vi "Init.vi"(8 "error in (no error)":errorcluster, 9 "Logging Root":path, 10 "VolatusAPI":refnum<class "VolatusAPI.lvclass">, 11 "EventHandlerTask in":refnum<class "EventHandlerTask.lvclass">) -> (0 "error out":errorcluster, 3 "EventHandlerTask out":refnum<class "EventHandlerTask.lvclass">)   [LabVIEW 2020, in "Volatus.lvlib" / "EventHandlerTask.lvclass"]
uses:
  EventHandlerTask.lvclass
  EventHandlerTask.lvclass/EventHandlerTask.ctl
  VolatusAPI/VolatusAPI.lvclass
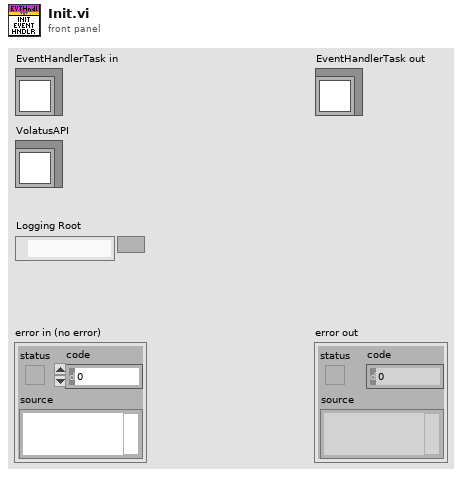
[diagram p1: front panel]
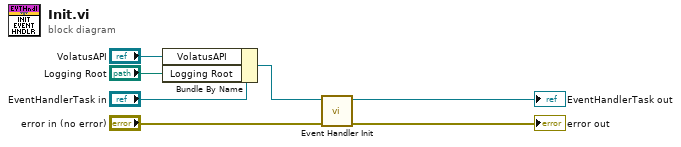
[diagram p0: block diagram]
diagram:
  n1 = Bundle By Name(cluster="EventHandlerTask in", "VolatusAPI"="VolatusAPI", "Logging Root"="Logging Root") -> (w2:refnum<class "EventHandlerTask.lvclass">)
  n2 = call-dynamic "Event Handler Init.vi"("error in (no error)"="error in (no error)", "EventHandlerTask in"=w2) -> ("error out"=→"error out":errorcluster, "EventHandlerTask out"=→"EventHandlerTask out":refnum<class "EventHandlerTask.lvclass">)  [unwired: 8 in]
